vi "parseUDPrequest.vi"(11 "data":string) -> (2 "value":string, 3 "command":string)   [LabVIEW 2017]
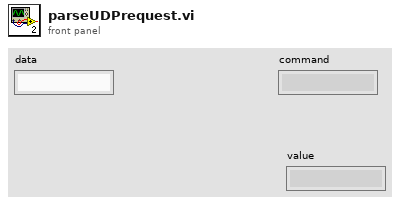
[diagram p1: front panel]
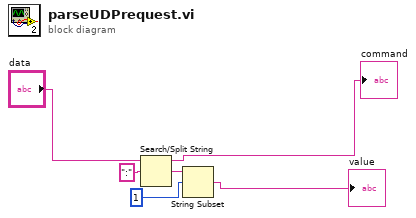
[diagram p0: block diagram]
diagram:
  n1 = Search/Split String(string="data", search string/char (-)=":") -> (substring before match=→"command":string, match + rest of string=w5:string)  [unwired: 1 in, 1 out]
  n2 = String Subset(string=w5, offset (0)=1) -> (substring=→"value":string)  [unwired: 1 in]
